vi "RANGE Delay ANSI Display.vi"(7 "Meter Number":T1, 8 "Error In":errorcluster, 9 "ANSI Start Time":dbl, 10 "Elapsed Time":dbl, 11 "DAQ Data Out in in":T2) -> (0 "Error Out":errorcluster, 2 "Display ANSI Average (BTU/hr) out":dbl, 3 "DAQ Data Out out":T2)   [LabVIEW 2016]
uses:
  Type Definitions/RANGE DAQ Data Four Meters.ctl
  Type Definitions/RANGE DAQ Data.ctl
  Drivers/Omega FMA-1600A Series Gas Flow Meter/Type Definitions/FMA1600A Gas Type.ctl
  Type Definitions/RANGE GAS Data.ctl
  Type Definitions/RANGE Panel Data.ctl
  Type Definitions/RANGE Meter Selector 1-2.ctl
  Type Definitions/Range Meter Bank.ctl
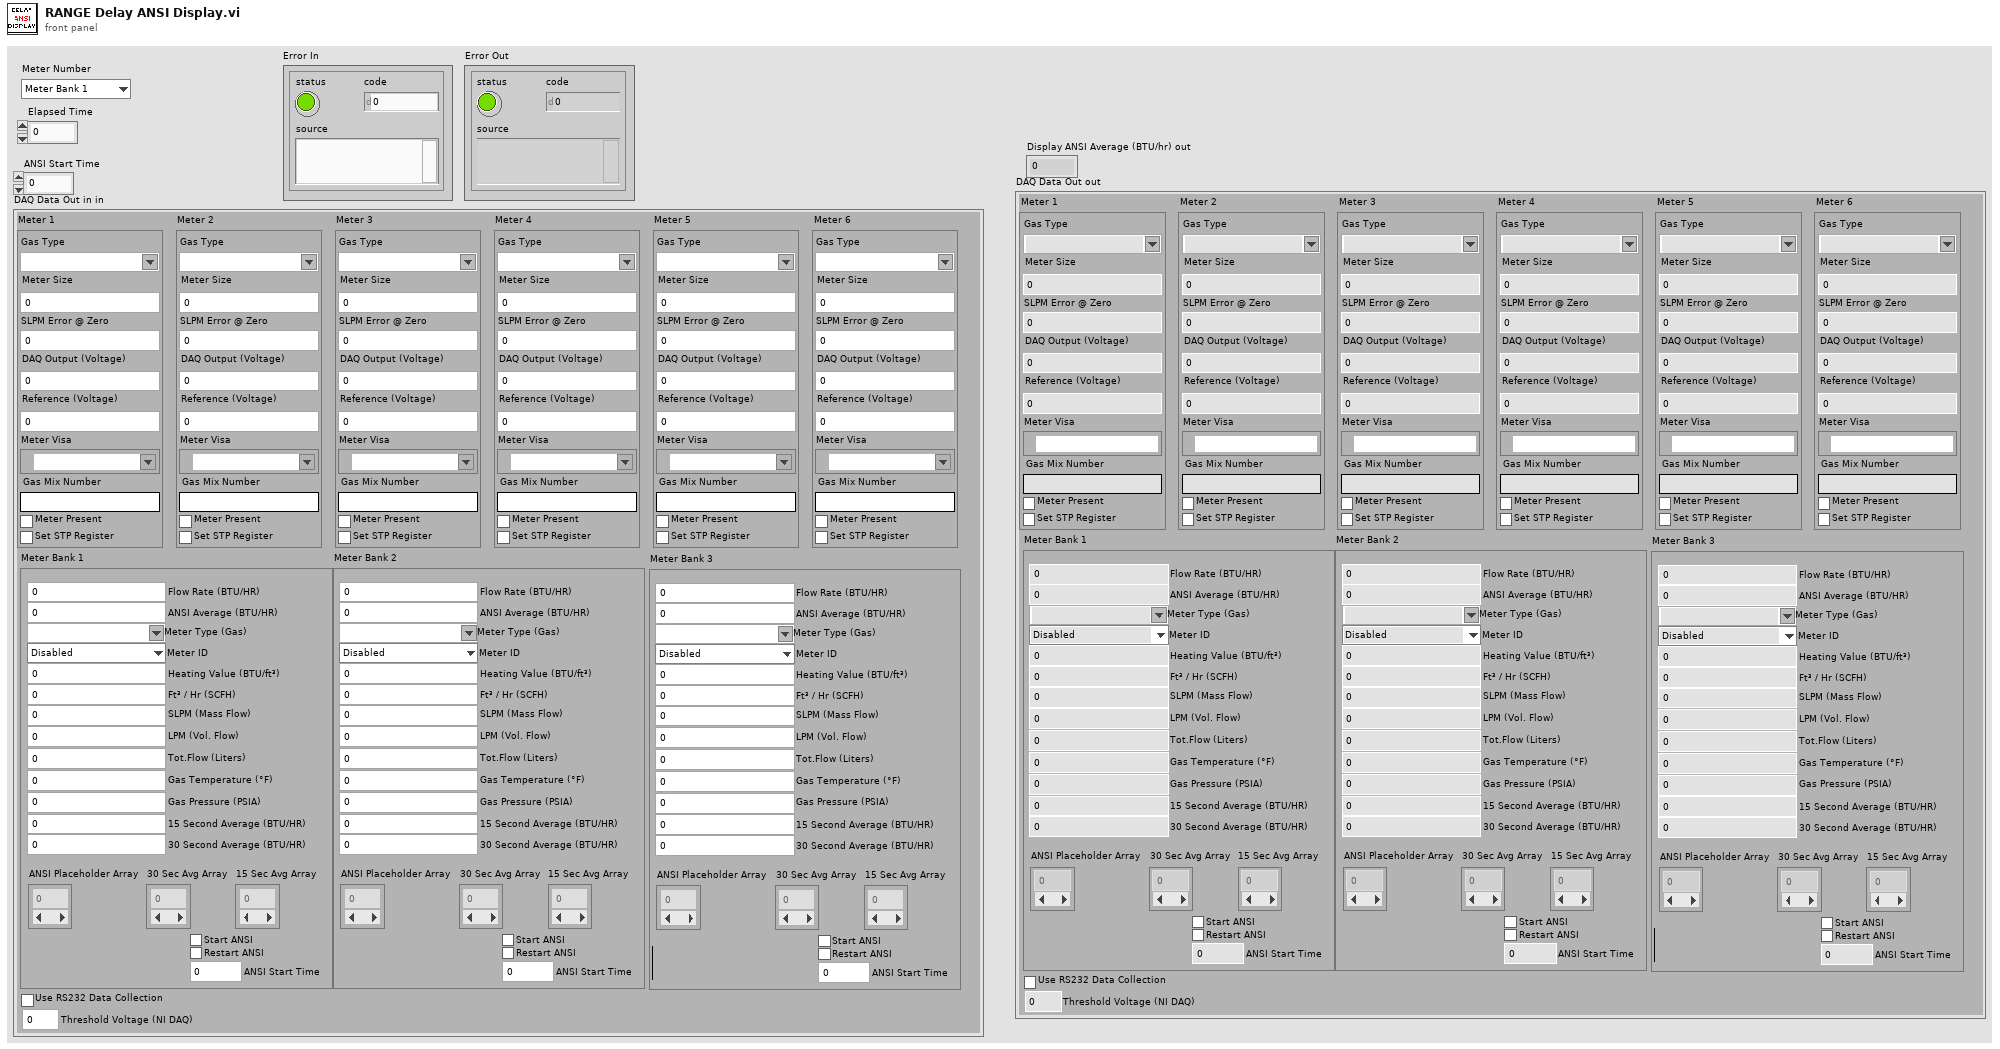
[diagram p1: front panel]
types:
  T1 = typedef "Range Meter Bank.ctl" = enum16{"Meter Bank 1", "Meter Bank 2", "Meter Bank 3"}
  T2 = typedef "RANGE DAQ Data Four Meters.ctl" = cluster{"Meter 1":T3, "Meter 2":T3, "Meter 3":T3, "Meter 4":T3, "Meter 5":T3, "Meter 6":T3, "Meter Bank 1":T5, "Meter Bank 2":T5, "Meter Bank 3":T5, "Threshold Voltage (NI DAQ)":dbl, "Use RS232 Data Collection":bool}
  T3 = typedef "RANGE DAQ Data.ctl" = cluster{"Meter Size":dbl, "DAQ Output (Voltage)":dbl, "Reference (Voltage)":dbl, "Meter Present":bool, "Meter Visa":refnum<visa-resource-name>, "Gas Type":T4, "SLPM Error @ Zero":dbl, "Gas Mix Number":string, "Set STP Register":bool}
  T4 = typedef "FMA1600A Gas Type.ctl" = string
  T5 = typedef "RANGE GAS Data.ctl" = cluster{"Flow Rate (BTU/HR)":dbl, "ANSI Placeholder Array":dbl[], "15 Sec Avg Array":dbl[], "30 Sec Avg Array ":dbl[], "ANSI Average (BTU/HR)":dbl, "Panel Data":T6, "Start ANSI":bool, "ANSI Start Time":dbl, "Restart ANSI":bool}
  T6 = typedef "RANGE Panel Data.ctl" = cluster{"Meter Type (Gas)":T4, "Meter ID":T7, "Heating Value (BTU/ft³)":dbl, "Ft³ / Hr (SCFH)":dbl, "15 Second Average (BTU/HR)":dbl, "30 Second Average (BTU/HR)":dbl, "SLPM (Mass Flow)":dbl, "LPM (Vol. Flow)":dbl, "Gas Temperature (°F)":dbl, "Gas Pressure (PSIA)":dbl, "Tot.Flow (Liters)":dbl}
  T7 = typedef "RANGE Meter Selector 1-2.ctl" = enum16{"Disabled", "Small", "Large"}
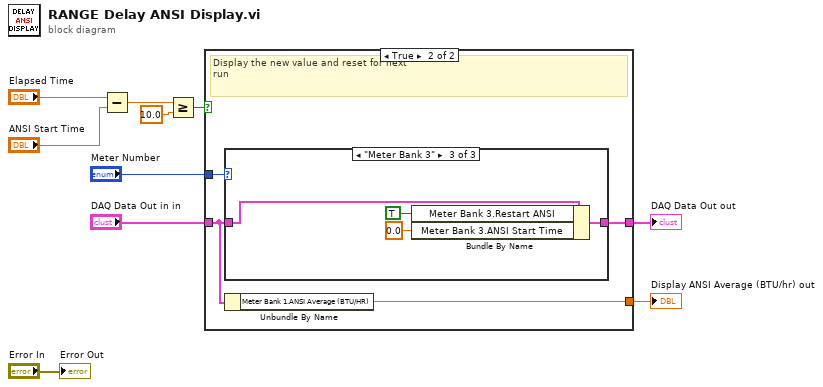
[diagram p0: block diagram]
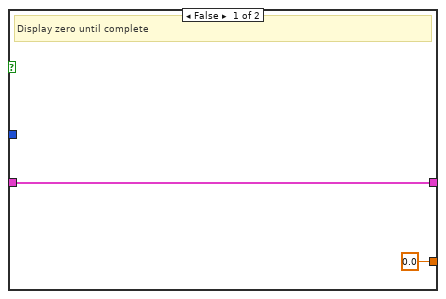
[diagram p2: hidden frame]
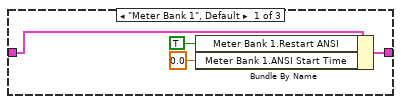
[diagram p3: hidden frame]
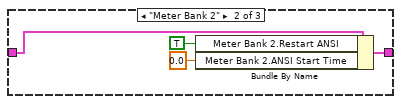
[diagram p4: hidden frame]
diagram:
  n1 = Subtract(x="Elapsed Time", y="ANSI Start Time") -> (x-y=w1:dbl)
  n2 = Greater Or Equal?(x=w1, y=10.0) -> (x >= y?=w5:bool)
  n3 = case shown="True" w5 {
    tunnel: "DAQ Data Out in in" -> [w12 w16]
    tunnel: [0.0 ("ANSI Average (BTU/HR)") w15] -> w9
    tunnel: [w12 w14] -> w10
    tunnel: "Meter Number" -> [_ w13]
    frame False {
      # "Display zero until complete"
    }
    frame True {
      # "Display the new value and reset for next \nrun"
      n4 = case shown="\"Meter Bank 3\"" w13 {
        tunnel: w16 -> [w20 w22 w27]
        tunnel: [w19 w23 w26] -> w14
        frame "Meter Bank 1", Default {
          n5 = Bundle By Name(cluster=w20, "Meter Bank 1.Restart ANSI"=TRUE, "Meter Bank 1.ANSI Start Time"=0.0) -> (w19:T2)
        }
        frame "Meter Bank 2" {
          n6 = Bundle By Name(cluster=w22, "Meter Bank 2.Restart ANSI"=TRUE, "Meter Bank 2.ANSI Start Time"=0.0) -> (w23:T2)
        }
        frame "Meter Bank 3" {
          n7 = Bundle By Name(cluster=w27, "Meter Bank 3.Restart ANSI"=TRUE, "Meter Bank 3.ANSI Start Time"=0.0) -> (w26:T2)
        }
      }
      n8 = Unbundle By Name(w16) -> ("Meter Bank 1.ANSI Average (BTU/HR)"=w15:dbl)
    }
  }
  "DAQ Data Out out" <- w10
  "Display ANSI Average (BTU/hr) out" <- w9
  "Error Out" <- "Error In"
